vi "NaN (SubVI).vi"() -> (3 "NaN":dbl)   [LabVIEW 2018, in "Application.lvlib"]
uses:
  Application.lvlib
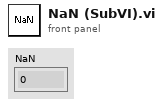
[diagram p1: front panel]
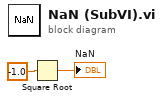
[diagram p0: block diagram]
diagram:
  n1 = Square Root(x=-1.0) -> (sqrt(x)=→"NaN":dbl)
